vi "Read All Data.vi"(7 "I2C Channel":u8, 8 "error in (no error)":errorcluster, 10 "Device Address":T8=104 items=["0x68"=104, "0x69"=105], 11 "LINX Resource":T1) -> (0 "error out":errorcluster, 1 "Gyro Data":T9, 2 "Accel Data":T9, 3 "LINX Resource":T1, 4 "Temperature (°C)":dbl)   [LabVIEW 2011, in "LVH-LINX.lvlib" / "MPU60X0.lvlib"]
doc: "Reads all data provided be the device."
uses:
  <vilib>/LabVIEW Hacker/LINX/Public/Sensors/Accelerometer/MPU60X0/MPU60X0.lvlib
  <vilib>/LabVIEW Hacker/LINX/Public/Sensors/Accelerometer/MPU60X0/DeviceAddresses.ctl
  <vilib>/LabVIEW Hacker/LINX/Private/Type Defs/LINX Ref.ctl
  <vilib>/LabVIEW Hacker/LINX/Private/Type Defs/Platform.ctl
  <vilib>/LabVIEW Hacker/LINX/Private/Type Defs/Interface.ctl
  <vilib>/LabVIEW Hacker/LINX/Private/Device/Type Defs/LINX Device Config.ctl
  <vilib>/LabVIEW Hacker/LINX/Private/Device/Type Defs/TCP Config.ctl
  <vilib>/LabVIEW Hacker/LINX/Private/Type Defs/Device Family.ctl
  <vilib>/LabVIEW Hacker/LINX/Private/Device/Type Defs/Channels.ctl
  <vilib>/LabVIEW Hacker/LINX/Public/Sensors/Accelerometer/MPU60X0/RegisterAddresses.ctl
  <vilib>/LabVIEW Hacker/LINX/LVH-LINX.lvlib
  <vilib>/LabVIEW Hacker/LINX/Private/Device/Device.lvlib
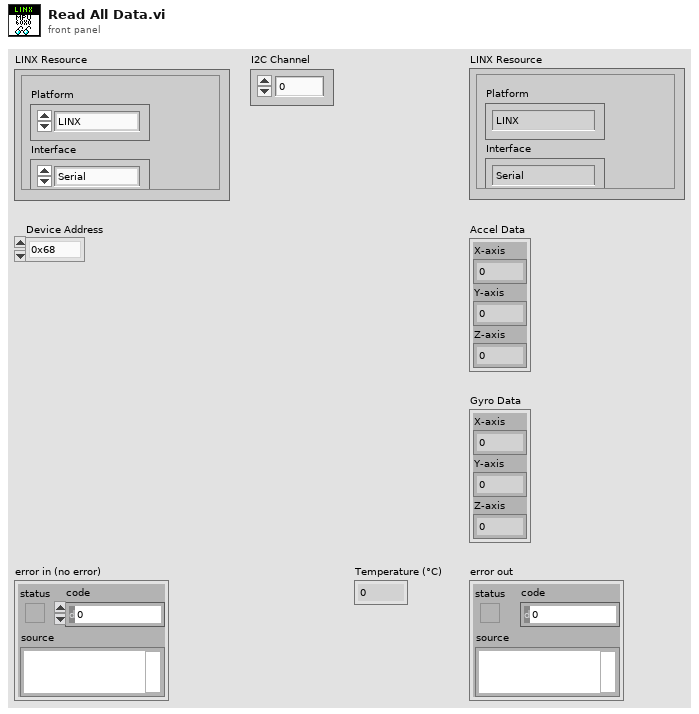
[diagram p1: front panel]
types:
  T1 = typedef "LVH-LINX.lvlib/LINX Ref.ctl" = cluster{"Platform":T2, "Interface":T3, "LINX Device Config":T4}
  T2 = typedef "LVH-LINX.lvlib/Platform.ctl" = enum16{"LINX", "myRIO"}
  T3 = typedef "LVH-LINX.lvlib/Interface.ctl" = enum16{"Serial", "TCP"}
  T4 = typedef "LVH-LINX.lvlib/Device.lvlib/LINX Device Config.ctl" = cluster{"Interface":T3, "COM Port":refnum<visa-resource-name>, "TCP Configuration":T5, "Device Family":T6, "Device ID":u8, "Device Name":string, "TCP Ref":refnum<k5>, "Channels":T7}
  T5 = typedef "LVH-LINX.lvlib/Device.lvlib/TCP Config.ctl" = cluster{"IP Address":string, "Port":u16}
  T6 = typedef "LVH-LINX.lvlib/Device Family.ctl" = enum8{"National Instruments", "Digilent", "Arduino"}
  T7 = typedef "LVH-LINX.lvlib/Channels.ctl" = cluster{"DI Channels":u8[], "DO Channels":u8[], "AI":u8[], "AO":u8[], "PWM":u8[], "QE":u8[], "UART":u8[], "I2C 2":u8[], "SPI":u8[], "CAN":u8[], "AI Ref (V)":dbl, "AO Resolution (Bits)":u8, "AO Ref (V)":dbl}
  T8 = typedef "LVH-LINX.lvlib/MPU60X0.lvlib/DeviceAddresses.ctl" = u8
  T9 = cluster{"X-axis":i16, "Y-axis":i16, "Z-axis":i16}
  T10 = typedef "LVH-LINX.lvlib/MPU60X0.lvlib/RegisterAddresses.ctl" = u16
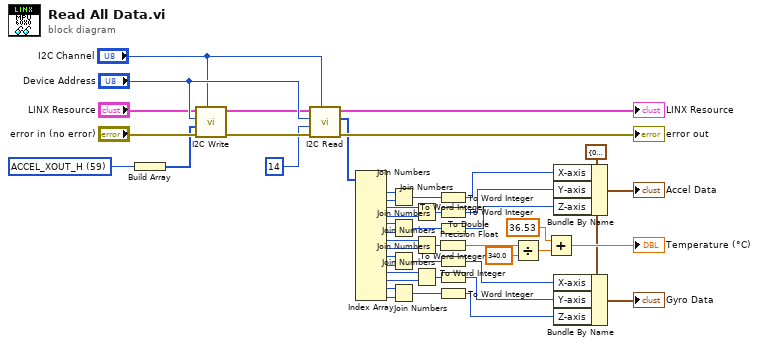
[diagram p0: block diagram]
diagram:
  w9 = T9 {"X-axis"=0, "Y-axis"=0, "Z-axis"=0} ("input cluster")
  w44 = T10 59 items=["SELF_TEST_X"=13, "SELF_TEST_Y"=14, "SELF_TEST_Z"=15, "SELF_TEST_A"=16, "SMPLRT_DIV"=25, "CONFIG"=26, "GYRO_CONFIG"=27, "ACCEL_CONFIG"=28, "MOT_THR"=31, "FIFO_EN"=35, "I2C_MST_CTRL"=36, "I2C_SLV0_ADDR"=37, "I2C_SLV0_REG"=38, "I2C_SLV0_CTRL"=39, "I2C_SLV1_ADDR"=40, "I2C_SLV1_REG"=41, "I2C_SLV1_CTRL"=42, "I2C_SLV2_ADDR"=43, "I2C_SLV2_REG"=44, "I2C_SLV2_CTRL"=45, "I2C_SLV3_ADDR"=46, "I2C_SLV3_REG"=47, "I2C_SLV3_CTRL"=48, "I2C_SLV4_ADDR"=49, "I2C_SLV4_REG"=50, "I2C_SLV4_DO"=51, "I2C_SLV4_CTRL"=52, "I2C_SLV4_DI"=53, "I2C_MST_STATUS"=54, "INT_PIN_CFG"=55, "INT_ENABLE"=56, "INT_STATUS"=58, "ACCEL_XOUT_H"=59, "ACCEL_XOUT_L"=60, "ACCEL_YOUT_H"=61, "ACCEL_YOUT_L"=62, "ACCEL_ZOUT_H"=63, "ACCEL_ZOUT_L"=64, "TEMP_OUT_H"=65, "TEMP_OUT_L"=66, "GYRO_XOUT_H"=67, "GYRO_XOUT_L"=68, "GYRO_YOUT_H"=69, "GYRO_YOUT_L"=70, "GYRO_ZOUT_H"=71, "GYRO_ZOUT_L"=72, "EXT_SENS_DATA_00"=73, "EXT_SENS_DATA_01"=74, "EXT_SENS_DATA_02"=75, "EXT_SENS_DATA_03"=76, "EXT_SENS_DATA_04"=77, "EXT_SENS_DATA_05"=78, "EXT_SENS_DATA_06"=79, "EXT_SENS_DATA_07"=80, "EXT_SENS_DATA_08"=81, "EXT_SENS_DATA_09"=82, "EXT_SENS_DATA_10"=83, "EXT_SENS_DATA_11"=84, "EXT_SENS_DATA_12"=85, "EXT_SENS_DATA_13"=86, "EXT_SENS_DATA_14"=87, "EXT_SENS_DATA_15"=88, "EXT_SENS_DATA_16"=89, "EXT_SENS_DATA_17"=90, "EXT_SENS_DATA_18"=91, "EXT_SENS_DATA_19"=92, "EXT_SENS_DATA_20"=93, "EXT_SENS_DATA_21"=94, "EXT_SENS_DATA_22"=95, "EXT_SENS_DATA_23"=96, "I2C_SLV0_DO"=99, "I2C_SLV1_DO"=100, "I2C_SLV2_DO"=101, "I2C_SLV3_DO"=102, "I2C_MST_DELAY_CTRL"=103, "SIGNAL_PATH_RESET"=104, "MOT_DETECT_CTRL"=105, "USER_CTRL"=106, "PWR_MGMT_1"=107, "PWR_MGMT_2"=108, "FIFO_COUNTH"=114, "FIFO_COUNTL"=115, "FIFO_R_W"=116, "WHO_AM_I"=117] ("Register Addresses")
  n1 = Build Array(w44) -> (w43:T10[])
  n2 = call <vilib>:"I2C Write.vi"("I2C Channel"="I2C Channel", "Error In"="error in (no error)", "Data"=w43, "I2C Slave Address (0)"="Device Address", "LINX Resource"="LINX Resource") -> ("Error Out"=w47:errorcluster, "LINX Resource"=w4:T1)  [unwired: 5 in]
  n3 = call <vilib>:"I2C Read.vi"("I2C Channel"="I2C Channel", "Error In"=w47, "Bytes To Read"=u8 14, "I2C Slave Address (0)"="Device Address", "LINX Resource"=w4) -> ("Error Out"=→"error out":errorcluster, "Data"=w40:u8[], "LINX Resource"=→"LINX Resource":T1)  [unwired: 4 in]
  n4 = Index Array(array=w40) -> (element #1=w39:u8, element #2=w38:u8, element #3=w37:u8, element #4=w36:u8, element #5=w35:u8, element #6=w34:u8, element #7=w33:u8, element #8=w32:u8, element #9=w31:u8, element #10=w30:u8, element #11=w29:u8, element #12=w28:u8, element #13=w27:u8, element #14=w26:u8)  [unwired: 14 in]
  n5 = Join Numbers(hi=w39, lo=w38) -> ((hi.lo)=w24:u16)
  n6 = Join Numbers(hi=w35, lo=w34) -> ((hi.lo)=w23:u16)
  n7 = Join Numbers(hi=w31, lo=w30) -> ((hi.lo)=w19:u16)
  n8 = Join Numbers(hi=w27, lo=w26) -> ((hi.lo)=w20:u16)
  n9 = Join Numbers(hi=w37, lo=w36) -> ((hi.lo)=w25:u16)
  n10 = Join Numbers(hi=w33, lo=w32) -> ((hi.lo)=w22:u16)
  n11 = Join Numbers(hi=w29, lo=w28) -> ((hi.lo)=w21:u16)
  n12 = To Word Integer(number=w24) -> (16bit integer=w13:i16)
  n13 = To Word Integer(number=w25) -> (16bit integer=w12:i16)
  n14 = To Word Integer(number=w23) -> (16bit integer=w11:i16)
  n15 = To Double Precision Float(number=w22) -> (double precision float=w18:dbl)
  n16 = To Word Integer(number=w19) -> (16bit integer=w8:i16)
  n17 = To Word Integer(number=w21) -> (16bit integer=w7:i16)
  n18 = To Word Integer(number=w20) -> (16bit integer=w6:i16)
  n19 = Divide(x=w18, y=340.0) -> (x/y=w16:dbl)
  n20 = Add(x=36.53, y=w16) -> (x+y=→"Temperature (°C)":dbl)
  n21 = Bundle By Name(cluster=w9, "X-axis"=w13, "Y-axis"=w12, "Z-axis"=w11) -> (→"Accel Data":T9)
  n22 = Bundle By Name(cluster=w9, "X-axis"=w8, "Y-axis"=w7, "Z-axis"=w6) -> (→"Gyro Data":T9)
